vi "PQ-12 (SubVI).vi"(2 "error in (no error)":errorcluster, 3 "Deploy / Retract [T/F]":bool) -> (0 "error out":errorcluster)   [LabVIEW 2018]
uses:
  <vilib>/Utility/error.llb/Error Cluster From Error Code.vi
  <vilib>/myRIO/Common/Instrument Driver Framework/myRIO v1.0/AI/vis/myRIO v1.0 Read AI.vi
  <vilib>/myRIO/Common/Instrument Driver Framework/myRIO v1.0/DIO/vis/myRIO v1.0 Write DIO.vi
  <vilib>/myRIO/Instrument Drivers/Onboard IO/AI/AI.lvlib
  <vilib>/myRIO/Instrument Drivers/Onboard IO/DIO/DIO.lvlib
panel:
  out "Values":dbl[](array[numeric])
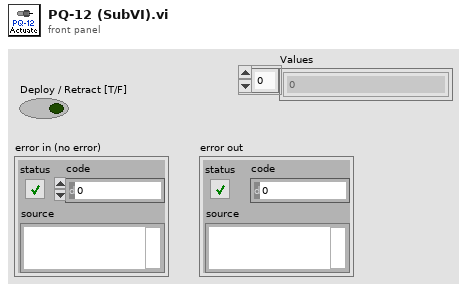
[diagram p1: front panel]
types:
  T1 = typedef "AI.lvlib/AI Reference.ctl" = cluster{"myRIO Reference":T2, "AI Channels List":T6, "AI Scaling Constants List":T8}
  T2 = typedef "myRIO Generic Hardware Reference.ctl" = cluster{"myRIO Model":T3, "myRIO Hardware Reference":T4}
  T3 = typedef "Hardware Version Enum.ctl" = enum16{"Unknown", "myRIO-1900", "myRIO-1950", "roboRIO", "NI ELVIS RIO CM", "ELVIS III"}
  T4 = typedef "myRIO v1.0 Reference.ctl" = cluster{"Generic FPGA Reference":T5, "Allow multiple opens":bool}
  T5 = typedef "Generic FPGA Reference.ctl" = refnum<k20>
  T6 = typedef "AI Channels List.ctl" = T7[]
  T7 = typedef "AI Channels Enum.ctl" = enum16{"Not Connected", "AudioIn/Left", "AudioIn/Right", "C/AI0", "C/AI1", "A/AI0", "A/AI1", "A/AI2", "A/AI3", "A/AI4", "A/AI5", "A/AI6", "A/AI7", "B/AI0", "B/AI1", "B/AI2", "B/AI3", "B/AI4", "B/AI5", "B/AI6", "B/AI7", "AI/AI0", "AI/AI1", "AI/AI2", "AI/AI3", "A/AI0 (DIFF)", "A/AI1 (DIFF)", "A/AI2 (DIFF)", "A/AI3 (DIFF)", "B/AI0 (DIFF)", "B/AI1 (DIFF)", "B/AI2 (DIFF)", "B/AI3 (DIFF)"}
  T8 = typedef "Analog Scaling Constants List.ctl" = T9[]
  T9 = typedef "Analog Scaling Constants.ctl" = cluster{"LSB Weight (Volts)":dbl, "Offset (Volts)":dbl, "Signed?":bool}
  T10 = typedef "DIO.lvlib/DIO Reference.ctl" = cluster{"myRIO Reference":T2, "DIO Channels List":T11}
  T11 = typedef "DIO Channels List.ctl" = T12[]
  T12 = typedef "DIO Channels Enum.ctl" = enum16{"Not Connected", "C/DIO0", "C/DIO1", "C/DIO2", "C/DIO3", "C/DIO4", "C/DIO5", "C/DIO6", "C/DIO7", "A/DIO0", "A/DIO1", "A/DIO2", "A/DIO3", "A/DIO4", "A/DIO5", "A/DIO6", "A/DIO7", "A/DIO8", "A/DIO9", "A/DIO10", "A/DIO11", "A/DIO12", "A/DIO13", "A/DIO14", "A/DIO15", "A/DIO16", "A/DIO17", "A/DIO18", "A/DIO19", "B/DIO0", "B/DIO1", "B/DIO2", "B/DIO3", "B/DIO4", "B/DIO5", "B/DIO6", "B/DIO7", "B/DIO8", "B/DIO9", "B/DIO10", "B/DIO11", "B/DIO12", "B/DIO13", "B/DIO14", "B/DIO15", "B/DIO16", "B/DIO17", "B/DIO18", "B/DIO19", "LED0", "LED1", "LED2", "LED3", "Button0", "DIO/DIO0", "DIO/DIO1", "DIO/DIO2", "DIO/DIO3", "DIO/DIO4", "DIO/DIO5", "DIO/DIO6", "DIO/DIO7", "DIO/DIO8", "DIO/DIO9", "SPI/CS0", "SPI/CS1", "SPI/CS2", "SPI/CS3", "LED RADIO (Green)", "LED RADIO (Red)", "LED COMM (Green)", "LED COMM (Red)", "LED MODE (Green)", "LED MODE (Red)"}
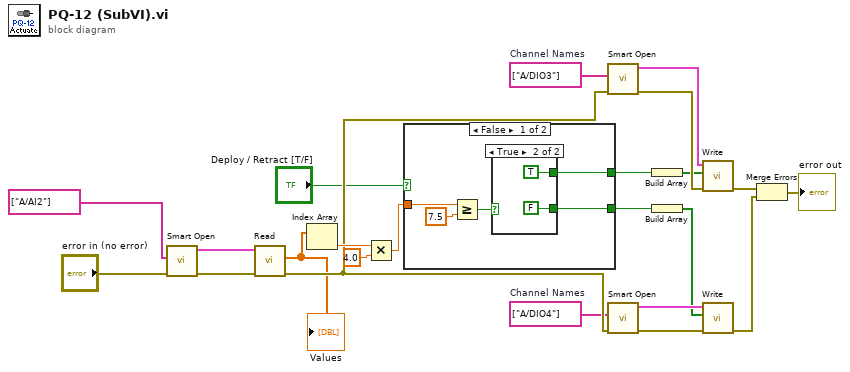
[diagram p0: block diagram]
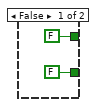
[diagram p2: hidden frame]
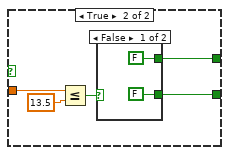
[diagram p3: hidden frame]
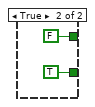
[diagram p4: hidden frame]
diagram:
  w14 = tag[] ["A/DIO3"]  # Channel Names
  w9 = tag[] ["A/DIO4"]  # Channel Names
  n1 = call <vilib>:"Smart Open.vi"("error in (no error)"="error in (no error)", "Channel Names"=tag[] ["A/AI2"]) -> ("error out"=w7:errorcluster, "AI Ref Out"=w6:T1)  [unwired: 8 in]
  n2 = call <vilib>:"Read.vi"("error in (no error)"=w7, "AI Ref In"=w6) -> ("error out"=w21:errorcluster, "Values"=w5:dbl[])  [unwired: 7 in, 1 out]
  "Values" <- w5
  n3 = Index Array(array=w5) -> (element=w23:dbl)  [unwired: 1 in]
  n4 = Multiply(x=w23, y=4.0) -> (x*y=w3:dbl)
  n5 = case shown="False" "Deploy / Retract [T/F]" {
    tunnel: [w28 w37] -> w13
    tunnel: [w27 w36] -> w18
    tunnel: w3 -> [w25 w34]
    frame False {
      n6 = Greater Or Equal?(x=w25, y=7.5) -> (x >= y?=w26:bool)
      n7 = case shown="True" w26 {
        tunnel: [FALSE FALSE] -> w28
        tunnel: [FALSE TRUE] -> w27
        frame False {
        }
        frame True {
        }
      }
    }
    frame True {
      n8 = Less Or Equal?(x=w34, y=13.5) -> (x <= y?=w35:bool)
      n9 = case shown="False" w35 {
        tunnel: [FALSE TRUE] -> w37
        tunnel: [FALSE FALSE] -> w36
        frame False {
        }
        frame True {
        }
      }
    }
  }
  n10 = call <vilib>:"Smart Open.vi"("error in (no error)"=w21, "Channel Names"=w14) -> ("error out"=w17:errorcluster, "DIO Ref Out"=w16:T10)  [unwired: 8 in]
  n11 = call <vilib>:"Smart Open.vi"("error in (no error)"=w21, "Channel Names"=w9) -> ("error out"=w12:errorcluster, "DIO Ref Out"=w11:T10)  [unwired: 8 in]
  n12 = Build Array(w18) -> (w15:bool[])
  n13 = Build Array(w13) -> (w10:bool[])
  n14 = call <vilib>:"Write.vi"("error in (no error)"=w17, "Values"=w15, "DIO Ref In"=w16) -> ("error out"=w19:errorcluster)  [unwired: 6 in, 1 out]
  n15 = call <vilib>:"Write.vi"("error in (no error)"=w12, "Values"=w10, "DIO Ref In"=w11) -> ("error out"=w20:errorcluster)  [unwired: 6 in, 1 out]
  n16 = Merge Errors(w19, w20) -> (→"error out":errorcluster)
